vi "create header.vi"(2 "Use Tab (T) ot Comma (F)":bool, 7 "EnableList":T1={"Cmd"=FALSE, "RegAdd"=FALSE, "Port"=FALSE, "Rsvd"=FALSE, "UTC"=FALSE, "Error"=FALSE, "Type"=FALSE, "NElements"=FALSE, "BitElementsColumn"=FALSE, "BitElementsAtTheEnd"=FALSE, "Read"=TRUE, "Write"=TRUE, "Event"=TRUE, "No Errors"=FALSE}) -> (8 "Line":string)   [LabVIEW 2010]
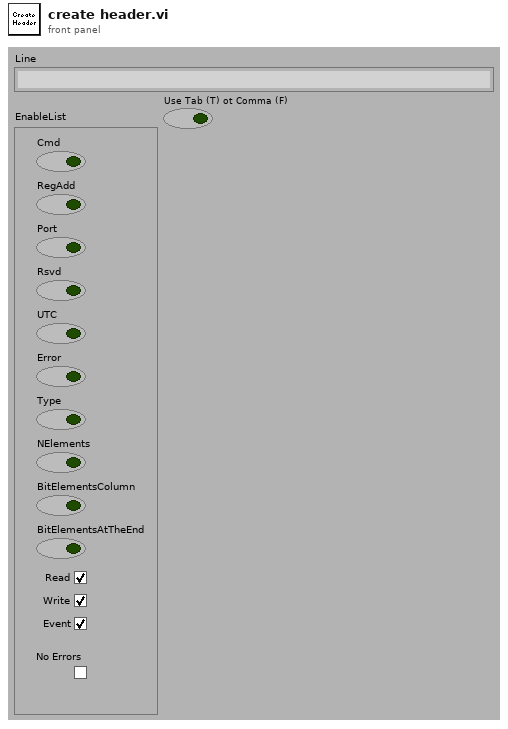
[diagram p1: front panel]
types:
  T1 = cluster{"Cmd":bool, "RegAdd":bool, "Port":bool, "Rsvd":bool, "UTC":bool, "Error":bool, "Type":bool, "NElements":bool, "BitElementsColumn":bool, "BitElementsAtTheEnd":bool, "Read":bool, "Write":bool, "Event":bool, "No Errors":bool}
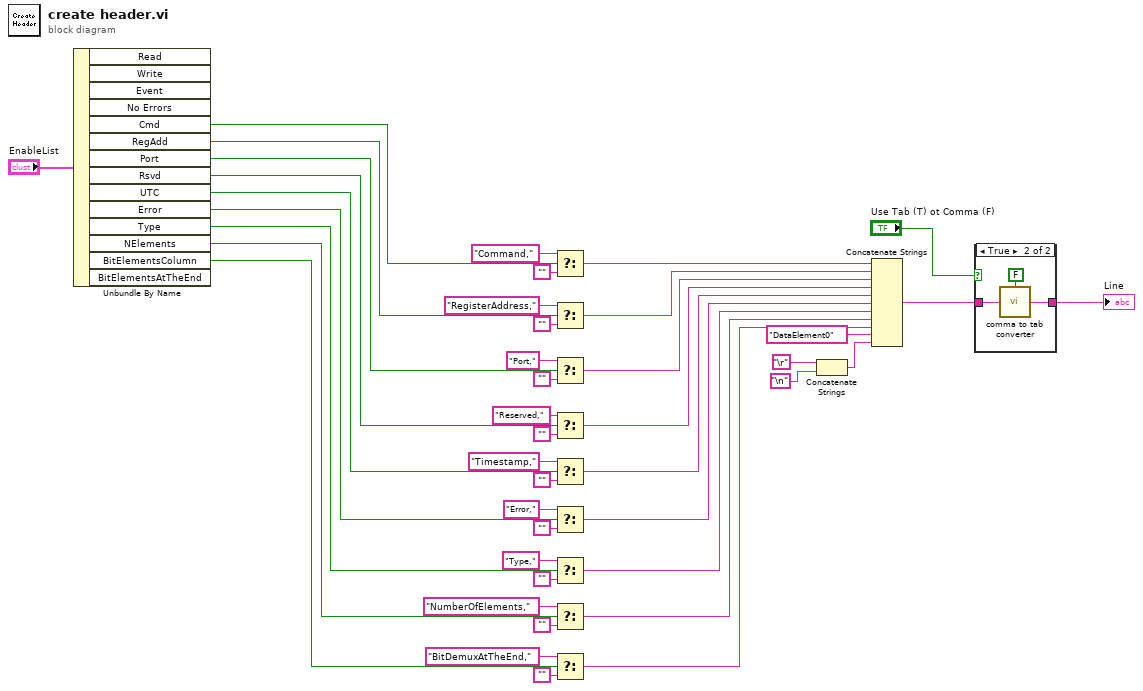
[diagram p0: block diagram]
diagram:
  n1 = Unbundle By Name("EnableList") -> ("Cmd"=w40:bool, "RegAdd"=w39:bool, "Port"=w16:bool, "Rsvd"=w37:bool, "UTC"=w13:bool, "Error"=w33:bool, "Type"=w31:bool, "NElements"=w29:bool, "BitElementsColumn"=w19:bool)  [unwired: 5 out]
  n2 = Select(t="Command,", s=w40, f="") -> (s? t:f=w28:string)
  n3 = Select(t="RegisterAddress,", s=w39, f="") -> (s? t:f=w21:string)
  n4 = Select(t="Port,", s=w16, f="") -> (s? t:f=w27:string)
  n5 = Select(t="Reserved," ("string"), s=w37, f="") -> (s? t:f=w26:string)
  n6 = Select(t="Timestamp,", s=w13, f="") -> (s? t:f=w25:string)
  n7 = Select(t="Error,", s=w33, f="") -> (s? t:f=w24:string)
  n8 = Select(t="Type,", s=w31, f="") -> (s? t:f=w23:string)
  n9 = Select(t="NumberOfElements,", s=w29, f="") -> (s? t:f=w22:string)
  n10 = Select(t="BitDemuxAtTheEnd,", s=w19, f="") -> (s? t:f=w8:string)
  n11 = Concatenate Strings("\r", "\n") -> (w4:string)
  n12 = Concatenate Strings(w28, w21, w27, w26, w25, w24, w23, w22, w8, "DataElement0" ("string"), w4) -> (w2:string)
  n13 = case shown="True" "Use Tab (T) ot Comma (F)" {
    tunnel: [w45 w48] -> w3
    tunnel: w2 -> [w45 w47]
    frame False {
    }
    frame True {
      n14 = call "comma to tab converter.vi"("System (T: system, F: period)"=FALSE, "',' string"=w47) -> ("'\\t' string"=w48:string)  [unwired: 13 in]
    }
  }
  "Line" <- w3
